vi "checkBeginBallChallengePlayVSS.vi"(8 "error in (no error)":errorcluster, 9 "last command_interpreted":T1, 10 "Game":refnum<class "Game.lvclass">, 11 "BallChallengePlayVSS in":refnum<class "BallChallengePlayVSS.lvclass">) -> (0 "error out":errorcluster, 2 "Boolean":bool, 3 "BallChallengePlayVSS out":refnum<class "BallChallengePlayVSS.lvclass">)   [LabVIEW 2023, in "BallChallengePlayVSS.lvclass"]
uses:
  BallChallengePlayVSS.lvclass
  Game_class/Game.lvclass
  Referee_class/command_interpreted.ctl
  Game_class/Game.lvclass/Game.ctl
  Referee_class/Referee.lvclass/Referee.ctl
  Game_class/Read Referee.vi
  Game_class/Read BallRef.vi
  Referee_class/Read command_interpreted.vi
  Referee_class/Referee.lvclass
  Ball_class/Ball.lvclass
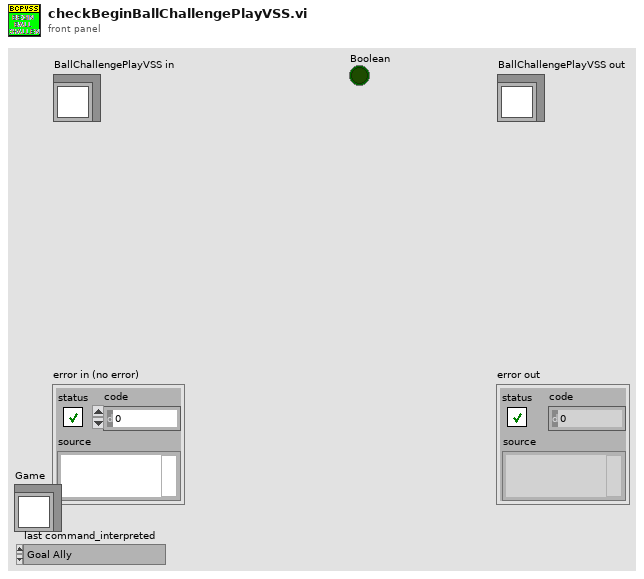
[diagram p1: front panel]
types:
  T1 = typedef "command_interpreted.ctl" = enum16{"Goal Ally", "Goal Enemy", "Ball Placement Enemy", "Ball Placement Ally", "Normal Half Time", "Extra Time  Break", "Extra Half Time", "None", "Post Game", "PKA Normal Start", "Prepare Kickoff Ally", "PKE Normal Start", "Prepare Kickoff Enemy", "Force Start", "Halt", "Timeout", "Prepare Penalty Ally", "Prepare Penalty Enemy", "PPA NormalStart", "PPE Normal Start", "Indirect Free Ally", "Direct Free Enemy", "Direct Free Ally", "Indirect Free Enemy", "Stop"}
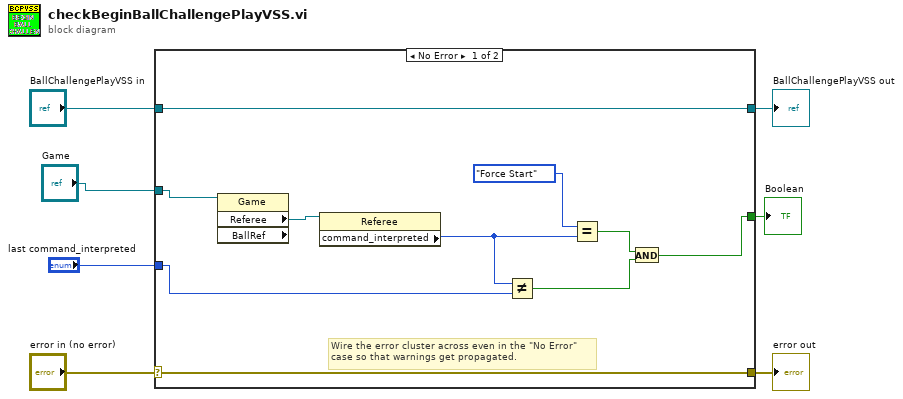
[diagram p0: block diagram]
diagram:
  n1 = case shown="No Error" "error in (no error)" {
    selector: "error in (no error)" -> [w16 w19]
    tunnel: [w16 w19] -> w6
    tunnel: [w17 w18] -> w4
    tunnel: "BallChallengePlayVSS in" -> [w17 w18]
    tunnel: "Game" -> [w10 _]
    tunnel: "last command_interpreted" -> [w9 _]
    tunnel: [w8 _] -> w1
    frame No Error {
      # "Wire the error cluster across even in the \"No Error\"\ncase so that warnings get propagated."
      n2 = property class="Game" props=["Referee", "BallRef"](reference=w10) -> ("Referee"=w15:refnum<class "Referee.lvclass">)  [unwired: 1 in, 3 out]
      n3 = property class="Referee"(reference=w15) -> ("command_interpreted"=w13:T1)  [unwired: 1 in, 2 out]
      n4 = Not Equal?(x=w13, y=w9) -> (x != y?=w11:bool)
      n5 = Equal?(x=command_interpreted."Force Start" ("command_interpreted"), y=w13) -> (x = y?=w12:bool)
      n6 = And(x=w12, y=w11) -> (x .and. y?=w8:bool)
    }
    frame Error {
    }
  }
  "error out" <- w6
  "BallChallengePlayVSS out" <- w4
  "Boolean" <- w1
